vi "Untitled 1.vi"   [LabVIEW 2013]
uses:
  classes/Tests/TestInterface/Tests.ctl
  classes/Devices/DeviceInterface/Devices.ctl
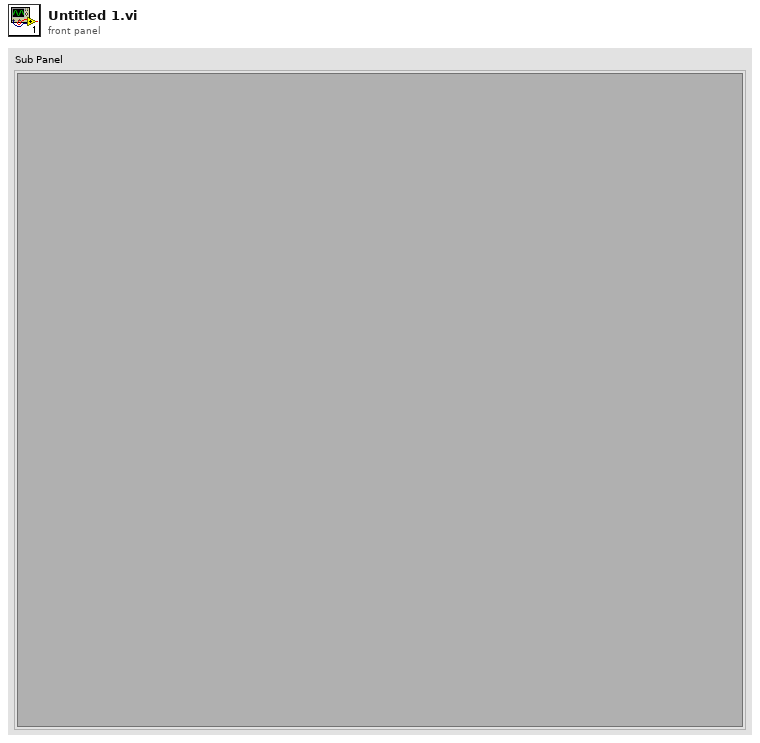
[diagram p1: front panel]
types:
  T1 = typedef "Devices.ctl" = enum16{"Tektronix RSA5106A", "emTestCWS500N", "CEG450"}
  T2 = typedef "Tests.ctl" = enum16{"Störaussendung", "Burst", "ESD", "Surge", "Spannungseinbruch", "HF-Felder"}
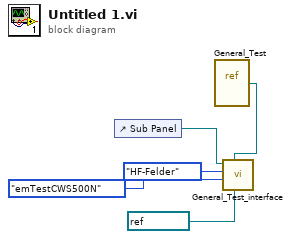
[diagram p0: block diagram]
diagram:
  n1 = control-ref of="Sub Panel"() -> (w3:refnum<vi>)
  n2 = vi-ref "General_Test.vi"() -> (w2:refnum<vi>)
  n3 = call "General_Test_interface.vi"("VISA resource name"=refnum<visa-resource-name> "COM5", "VI Refnum"=w2, "device"=Devices."emTestCWS500N", "test"=Tests."HF-Felder", "SubPanel in"=w3) -> ()  [unwired: 2 in, 5 out]
